vi "Client.vi"() -> ()   [LabVIEW 2021, in "Unary.lvlib"]
uses:
  Unary.lvlib
  TypeDef/I2C_Bus_Timing.ctl
  TypeDef/Pin_Levels.ctl
  Demo_client/RPC Messages/Communication_ActionReply.ctl
  Demo_client/RPC Messages/Communication_ActionRequest.ctl
  cbfacbe5-3d9c-4496-8a1c-3cba7c06b08e.vi
  7081ad6e-fbdd-4988-885d-712b26b53869.vi
  a666b6d7-ce01-4b70-acb0-9b8800d8cd6e.vi
  <vilib>/JDP Science/JSONtext/Variant to JSON Text.vi
  <vilib>/JDP Science/JSONtext/JSON text to Variant.vi
  <vilib>/JDP Science/JSONtext/LVClass Serializer/JSONtext LVClass Serializer.lvclass
  Demo_client/Demo_client.lvlib
panel:
  in  "gRPC Address":string="localhost:50051"
  out "I2C Pin Levels Response":T1={"Reply"="I2C Pin Levels", "Status"="Pass"}
  out "Configure I2C Bus timing Response":T1={"Reply"="Configure I2C Bus timing", "Status"="Pass"}
  in  "I2C Pin Levels":T2={"SCL VIH (V)"=1.8, "SCL VIL (V)"=1.8, "SCL Load Current (A)"=0.0015, "SDA VIH (V)"=0.0, "SDA VIL (V)"=0.0, "SDA Load Current (A)"=0.0015, "ModSeIL Termination Mode"="Internal", "ModSeIL VIL (V)"=0.0, "ModSeIL VIH (V)"=1.8} {"ModSeIL VIH (V)" min=-2.0 max=6.0 step=0.1 format="%#_2g"; "ModSeIL VIL (V)" min=-2.0 max=6.0 step=0.1 format="%#_2g"; "SDA Load Current (A)" min=0.0015 max=0.024 step=0.001 format="%#_2p"; "SDA VIH (V)" min=-2.0 max=6.0 step=0.1 format="%#_3g"; "SDA VIL (V)" min=-2.0 max=6.0 step=0.1 format="%#_3g"; "SCL Load Current (A)" min=0.0015 max=0.024 step=0.001 format="%#_2p"; "SCL VIH (V)" min=-2.0 max=6.0 step=0.1 format="%#_3g"; "SCL VIL (V)" min=-2.0 max=6.0 step=0.1 format="%#_3g"}
  in  "Configure I2C Bus timing":T3={"Frequency(Hz)"=1000000.0, "T_HIGH(ns)"=500.0, "T_LOW(ns)"=250.0, "T_SU_STO(ns)"=250.0, "T_SU_STA(ns)"=500.0, "T_SU_DAT(ns)"=250.0, "T_BUF(ns)"=250.0, "T_HD_STA(ns)"=250.0, "T_HD_DAT(ns)"=250.0} {"Frequency(Hz)" min=10000.0 max=25000000.0 step=100.0 format="%#_6p"; "T_HD_DAT(ns)" step=1.0 format="%#_5g"; "T_SU_STA(ns)" min=0.0 step=1.0 format="%#_5g"; "T_HD_STA(ns)" min=0.0 step=1.0 format="%#_5g"; "T_SU_STO(ns)" min=0.0 step=1.0 format="%#_5g"; "T_BUF(ns)" min=0.0 step=1.0 format="%#_5g"; "T_HIGH(ns)" min=0.0 step=1.0 format="%#_5g"; "T_LOW(ns)" min=0.0 step=1.0 format="%#_5g"; "T_SU_DAT(ns)" step=1.0 format="%#_5g"}
  # "Unary Client"
  # "Pin Levels Configuration"
  # "SCL"
  # "SDA"
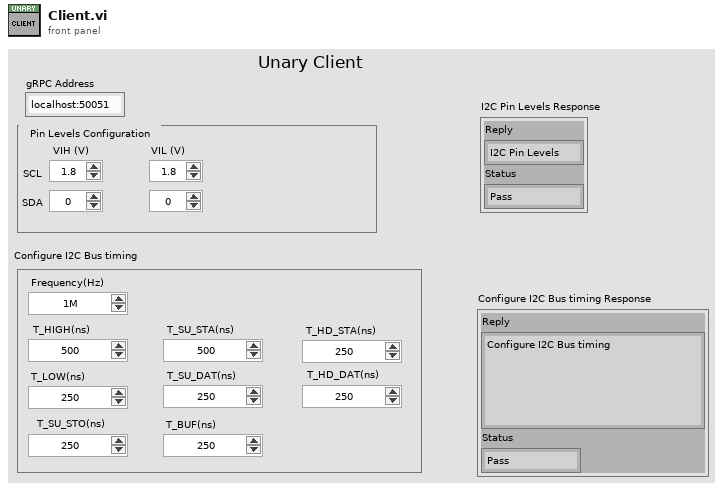
[diagram p1: front panel]
types:
  T1 = typedef "Demo_client.lvlib/Communication_ActionReply.ctl" = cluster{"Reply":string, "Status":string}
  T2 = typedef "Unary.lvlib/Pin_Levels.ctl" = cluster{"SCL VIH (V)":dbl, "SCL VIL (V)":dbl, "SCL Load Current (A)":dbl, "SDA VIH (V)":dbl, "SDA VIL (V)":dbl, "SDA Load Current (A)":dbl, "ModSeIL Termination Mode":string, "ModSeIL VIL (V)":dbl, "ModSeIL VIH (V)":dbl}
  T3 = typedef "Unary.lvlib/I2C_Bus_Timing.ctl" = cluster{"Frequency(Hz)":dbl, "T_HIGH(ns)":dbl, "T_LOW(ns)":dbl, "T_SU_STO(ns)":dbl, "T_SU_STA(ns)":dbl, "T_SU_DAT(ns)":dbl, "T_BUF(ns)":dbl, "T_HD_STA(ns)":dbl, "T_HD_DAT(ns)":dbl}
  T4 = typedef "grpc-lvsupport-release.lvlib/grpcId.ctl" = u64
  T5 = typedef "Demo_client.lvlib/Communication_ActionRequest.ctl" = cluster{"Request":string, "Data":string}
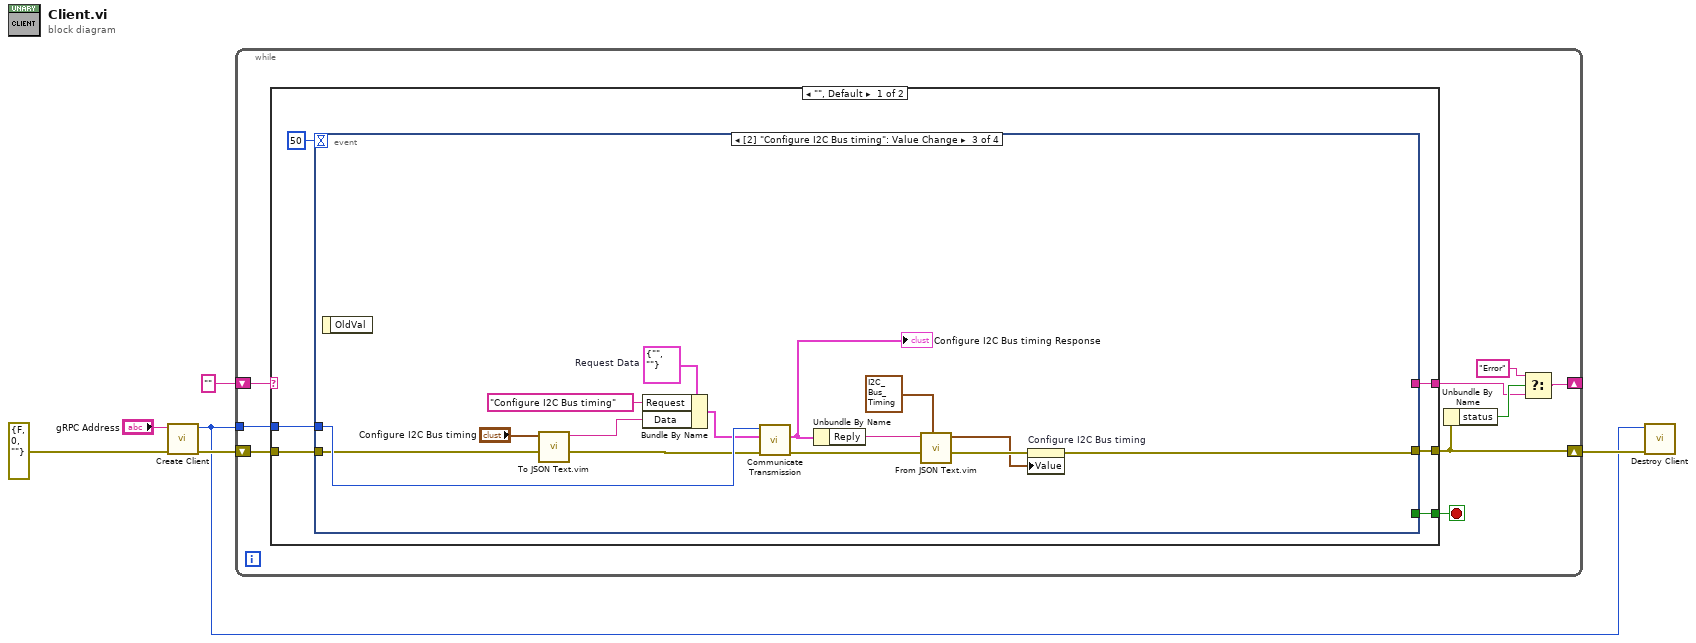
[diagram p0: block diagram]
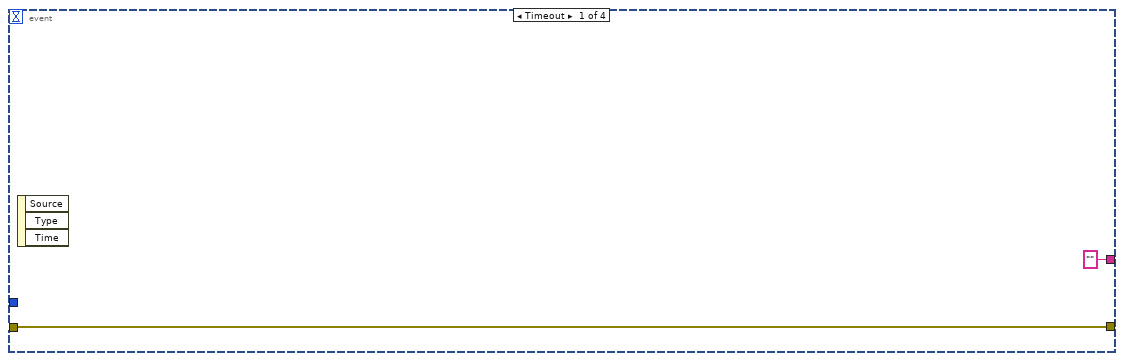
[diagram p2: hidden frame]
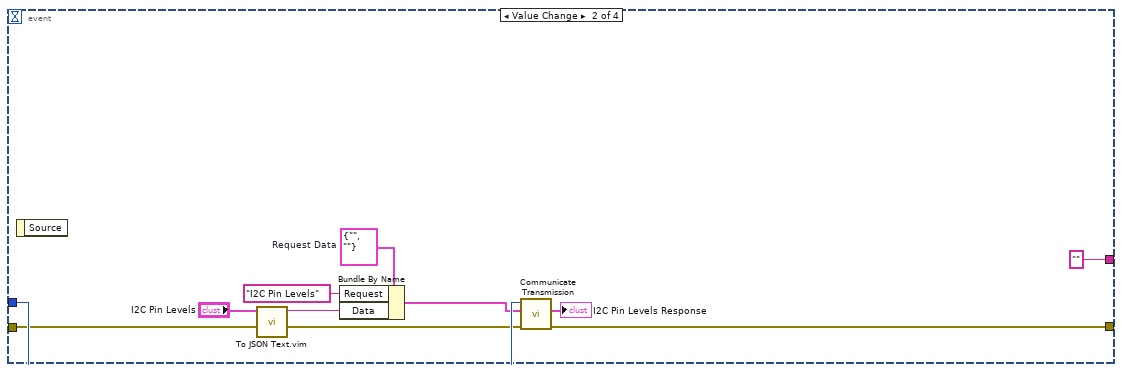
[diagram p3: hidden frame]
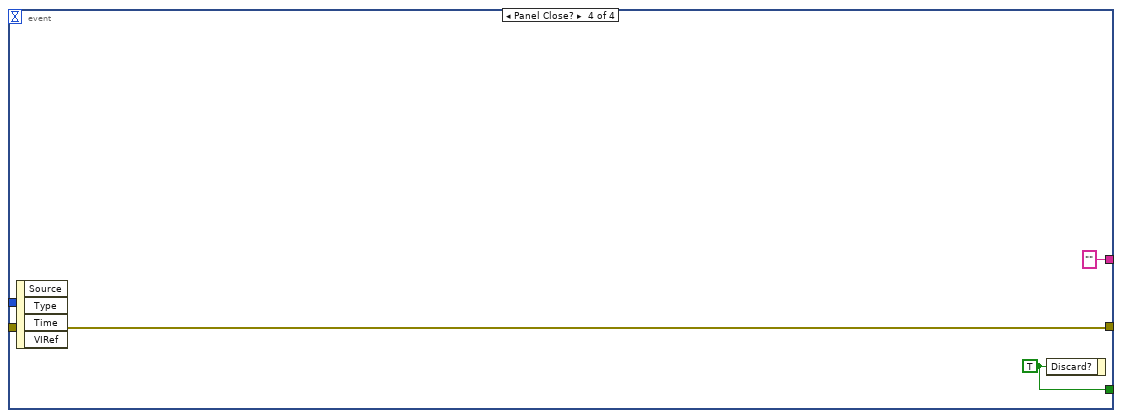
[diagram p4: hidden frame]
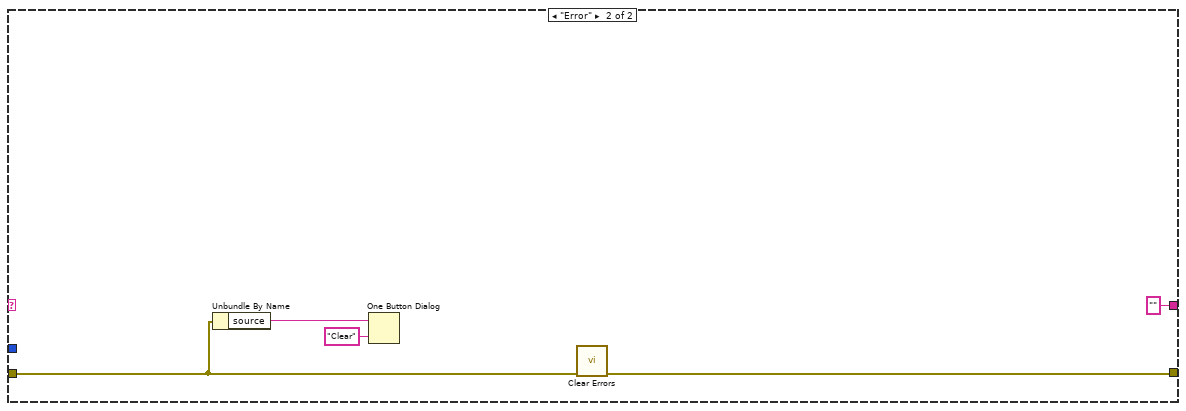
[diagram p5: hidden frame]
diagram:
  n1 = call "Create Client.vi"("error in"=errorcluster {"status"=FALSE, "code"=0, "source"=""} ("error in (no error)"), "address"="gRPC Address") -> ("error out"=w5:errorcluster, "gRPC ID Out"=w1:T4)  [unwired: 8 in]
  n2 = while {
    shift-right: [w11] -> w2
    shift-left: w5 -> [w14]
    tunnel: w1 -> [w13]
    shift-right: [w9] -> _
    shift-left: "" -> [w15]
    stop <- w12 stop-if-true
    n3 = case shown="\"\", Default" w15 {
      tunnel: w14 -> [w21 w56]
      tunnel: [w20 w57] -> w11
      tunnel: w13 -> [w19 _]
      tunnel: [w18 ""] -> w8
      tunnel: [w17 _] -> w12
      frame "", Default {
        n4 = event shown="[2] \"Configure I2C Bus timing\": Value Change" {
          selector: _ -> [_ _ _ _]
          dyn-events: _ -> [_ _ _ _]
          timeout: 50 -> [_ _ _ _]
          tunnel: w21 -> [w23 w26 w42 w52]
          tunnel: [w23 w33 w45 w52] -> w20
          tunnel: w19 -> [_ w32 w48 _]
          tunnel: ["" "" _ ""] -> w18
          tunnel: [_ _ _ w50] -> w17
          event Timeout {
            n5 = event-data() -> ()  [unwired: 1 in, 3 out]
          }
          event Value Change {
            w31 = T5 {"Request"="", "Data"=""}  # Request Data
            n6 = event-data() -> ()  [unwired: 1 in, 1 out]
            n7 = call "To JSON Text.vim"("error in (no error)"=w26, "Anything"="I2C Pin Levels") -> ("error out"=w27:errorcluster, "<JSON>"=w24:string)  [unwired: 8 in]
            n8 = Bundle By Name(cluster=w31, "Request"="I2C Pin Levels", "Data"=w24) -> (w29:T5)
            n9 = call "Communicate Transmission.vi"("error in"=w27, "Request Data"=w29, "gRPC ID"=w32) -> ("error out"=w33:errorcluster, "Response Data"=→"I2C Pin Levels Response":T1)  [unwired: 6 in, 1 out]
          }
          event Value Change {
            w46 = T5 {"Request"="", "Data"=""}  # Request Data
            n10 = event-data() -> ()  [unwired: 1 in, 1 out]
            n11 = call "To JSON Text.vim"("error in (no error)"=w42, "Anything"="Configure I2C Bus timing") -> ("error out"=w43:errorcluster, "<JSON>"=w40:string)  [unwired: 8 in]
            n12 = Bundle By Name(cluster=w46, "Request"="Configure I2C Bus timing", "Data"=w40) -> (w47:T5)
            n13 = call "Communicate Transmission.vi"("error in"=w43, "Request Data"=w47, "gRPC ID"=w48) -> ("error out"=w39:errorcluster, "Response Data"=w44:T1)  [unwired: 6 in, 1 out]
            "Configure I2C Bus timing Response" <- w44
            n14 = Unbundle By Name(w44) -> ("Reply"=w37:string)
            n15 = call "From JSON Text.vim"("Data Type and Default Value"=T3 {"Frequency(Hz)"=1000000.0, "T_HIGH(ns)"=500.0, "T_LOW(ns)"=250.0, "T_SU_STO(ns)"=250.0, "T_SU_STA(ns)"=500.0, "T_SU_DAT(ns)"=250.0, "T_BUF(ns)"=250.0, "T_HD_STA(ns)"=250.0, "T_HD_DAT(ns)"=250.0} ("Configure I2C Bus timing"), "error in (no error)"=w39, "JSON"=w37) -> ("error out"=w38:errorcluster, "Data out"=w35:T3)  [unwired: 7 in]
            n16 = property on="Configure I2C Bus timing" class="Clust (strict)"(error in=w38, "Value"=w35) -> (error out=w45:errorcluster)  [unwired: 1 in, 1 out]
          }
          event Panel Close? {
            w50 = TRUE ("Discard?")
            n17 = event-data() -> ()  [unwired: 1 in, 4 out]
            n18 = event-data("Discard?"=w50) -> ()  [unwired: 1 in, 1 out]
          }
        }
      }
      frame "Error" {
        n19 = Unbundle By Name(w56) -> ("source"=w54:string)
        n20 = One Button Dialog(message=w54, button name ("OK")="Clear") -> ()  [unwired: 1 out]
        n21 = call <vilib>:"Clear Errors.vi"("error in (no error)"=w56) -> ("error out"=w57:errorcluster)  [unwired: 5 in, 1 out]
      }
    }
    n22 = Unbundle By Name(w11) -> ("status"=w10:bool)
    n23 = Select(t="Error", s=w10, f=w8) -> (s? t:f=w9:string)
  }
  n24 = call "Destroy Client.vi"("error in"=w2, "gRPC ID"=w1) -> ()  [unwired: 9 in, 1 out]
